vi "EnableDisableControls(SubVI).vi"(7 "Enabled ?":T1(ring), 8 "error in (no error)":errorcluster, 11 "References Array":refnum<vi>[](array[refnum])) -> (0 "error out":errorcluster)   [LabVIEW 2018, in "MainFrameLib.lvlib"]
uses:
  MainFrameLib.lvlib
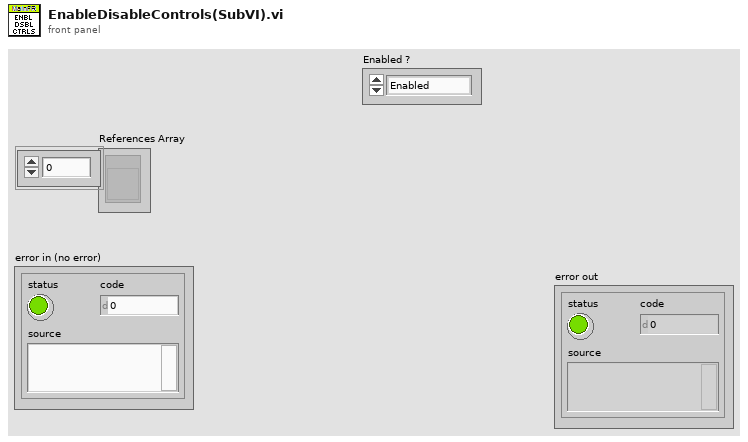
[diagram p1: front panel]
types:
  T1 = enum8{"Enabled", "Disabled", "Disabled and Grayed Out"}
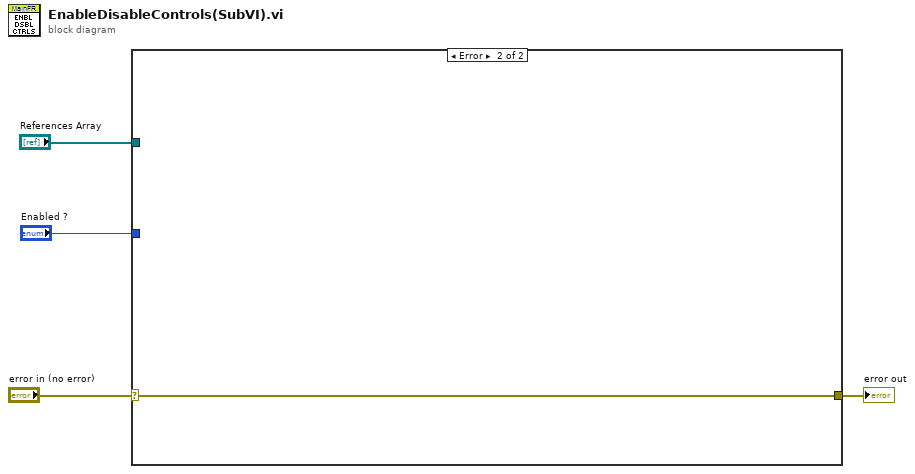
[diagram p0: block diagram]
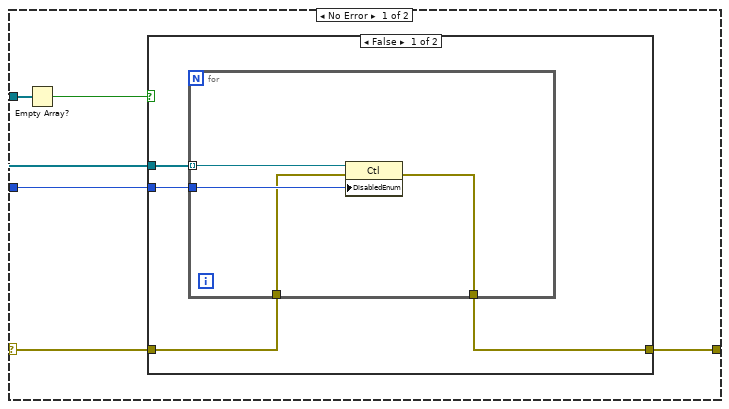
[diagram p2: hidden frame]
diagram:
  n1 = case shown="Error" "error in (no error)" {
    selector: "error in (no error)" -> [w5 w19]
    tunnel: "References Array" -> [w8 _]
    tunnel: "Enabled ?" -> [w7 _]
    tunnel: [w6 w19] -> w2
    frame No Error {
      n2 = Empty Array?(array=w8) -> (empty?=w9:bool)
      n3 = case shown="False" w9 {
        tunnel: w8 -> [w13 _]
        tunnel: w7 -> [w12 _]
        tunnel: w5 -> [w11 w18]
        tunnel: [w10 w18] -> w6
        frame False {
          n4 = for {
            tunnel: w13 -> [w17] mode=indexing
            tunnel: w12 -> [w16]
            tunnel: w11 -> [w15]
            tunnel: [w14] -> w10
            n5 = property class="Ctl"(reference=w17, error in=w15, "DisabledEnum"=w16) -> (error out=w14:errorcluster)  [unwired: 1 out]
          }
        }
        frame True {
        }
      }
    }
    frame Error {
    }
  }
  "error out" <- w2
